vi "add_ROI.vi"(8 "error in (no error)":errorcluster, 10 "roi":refnum<class "RoiGeneric.lvclass">, 11 "RoiCollection in":refnum<class "RoiCollection.lvclass">) -> (0 "error out":errorcluster, 3 "RoiCollection out":refnum<class "RoiCollection.lvclass">)   [LabVIEW 2010, in "RoiCollection.lvclass"]
uses:
  RoiCollection.lvclass
  RoiGeneric/RoiGeneric.lvclass
  RoiCollection.lvclass/RoiCollection.ctl
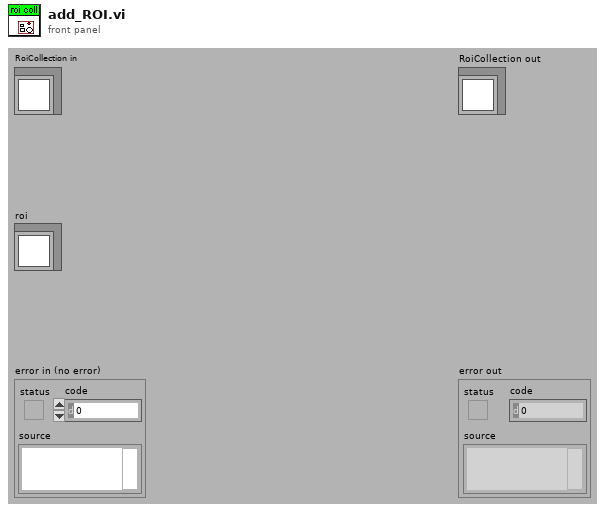
[diagram p1: front panel]
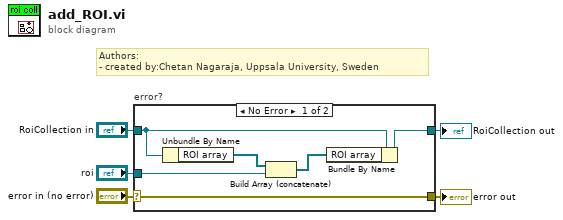
[diagram p0: block diagram]
diagram:
  # "Authors: \n- created by:Chetan Nagaraja, Uppsala University, Sweden"
  n1 = case "error?" shown="No Error" "error in (no error)" {
    selector: "error in (no error)" -> [w11 w13]
    tunnel: [w11 w13] -> w4
    tunnel: [w7 w12] -> w2
    tunnel: "RoiCollection in" -> [w6 w12]
    tunnel: "roi" -> [w10 _]
    frame No Error {
      n2 = Unbundle By Name(w6) -> ("ROI array"=w9:refnum<class "RoiGeneric.lvclass">[])
      n3 = Build Array (concatenate)(w9, w10) -> (w8:refnum<class "RoiGeneric.lvclass">[])
      n4 = Bundle By Name(cluster=w6, "ROI array"=w8) -> (w7:refnum<class "RoiCollection.lvclass">)
    }
    frame Error {
    }
  }
  "error out" <- w4
  "RoiCollection out" <- w2
